vi "roboRIO v1.0 Reserve Timer IRQ.vi"(4 "Callback VI Ref":T1, 5 "Allow Overwrite?":bool, 7 "Reserve?":bool, 8 "error in (no error)":errorcluster, 10 "Interval(us)":u32, 11 "Timer ID":u8) -> (0 "error out":errorcluster, 2 "Succeed?":bool)   [LabVIEW 2021]
uses:
  <vilib>/myRIO/Common/Instrument Driver Framework/myRIO v1.0/IRQ/typedefs/Callback VI Ref.ctl
  <vilib>/myRIO/Common/Instrument Driver Framework/Utilities/typedefs/FPGA Ref Manager Action Enum.ctl
  <vilib>/myRIO/Common/Instrument Driver Framework/myRIO v1.0/IRQ/typedefs/Timer IRQ.ctl
  <vilib>/myRIO/Common/Instrument Driver Framework/myRIO v1.0/IRQ/typedefs/IO IRQ Channels Enum.ctl
  <vilib>/myRIO/Common/Instrument Driver Framework/myRIO v1.0/IRQ/typedefs/IRQ Type.ctl
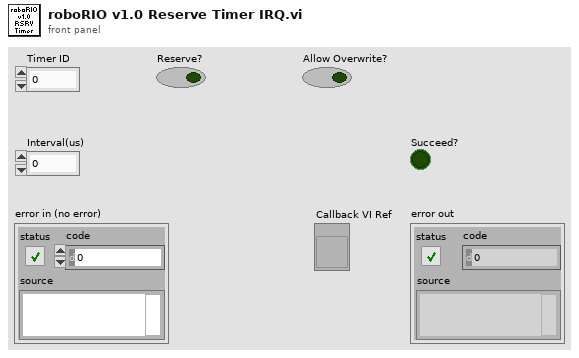
[diagram p1: front panel]
types:
  T1 = typedef "Callback VI Ref.ctl" = refnum<vi>
  T2 = typedef "FPGA Ref Manager Action Enum.ctl" = enum16{"Get", "Set", "Reset"}
  T3 = typedef "Timer IRQ.ctl" = cluster{"Remaining(us)":u32, "Timer ID":u8, "Interval(us)":u32, "Callback VI Ref":T1, "Allow Overwrite?":bool, "Timer enabled?":bool}
  T4 = typedef "IO IRQ Channels Enum.ctl" = enum16{"Not Connected", "A/AI0 (Interrupt)", "A/AI1 (Interrupt)", "A/DIO0 (Interrupt)", "A/DIO1 (Interrupt)", "A/DIO2 (Interrupt)", "A/DIO3 (Interrupt)", "Button0 (Interrupt)", "B/AI0 (Interrupt)", "B/AI1 (Interrupt)", "B/DIO0 (Interrupt)", "B/DIO1 (Interrupt)", "B/DIO2 (Interrupt)", "B/DIO3 (Interrupt)"}
  T5 = typedef "IRQ Type.ctl" = enum16{"Timer", "Analog falling edge", "Analog rising edge", "Digital falling edge", "Digital rising edge", "Digital edge"}
  T6 = typedef "Timer IRQ Array.ctl" = T3[]
  T7 = typedef "Generic FPGA Reference.ctl" = refnum<k20>
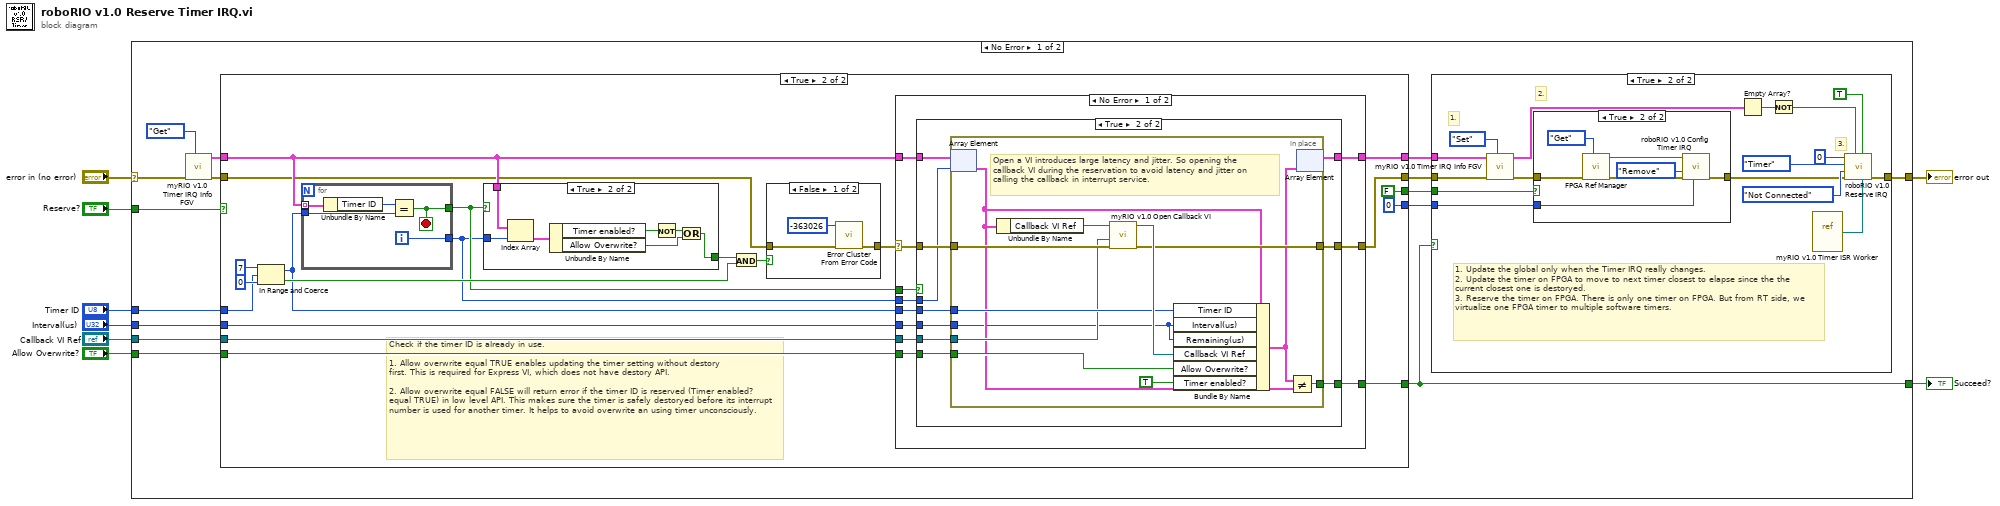
[diagram p0: block diagram]
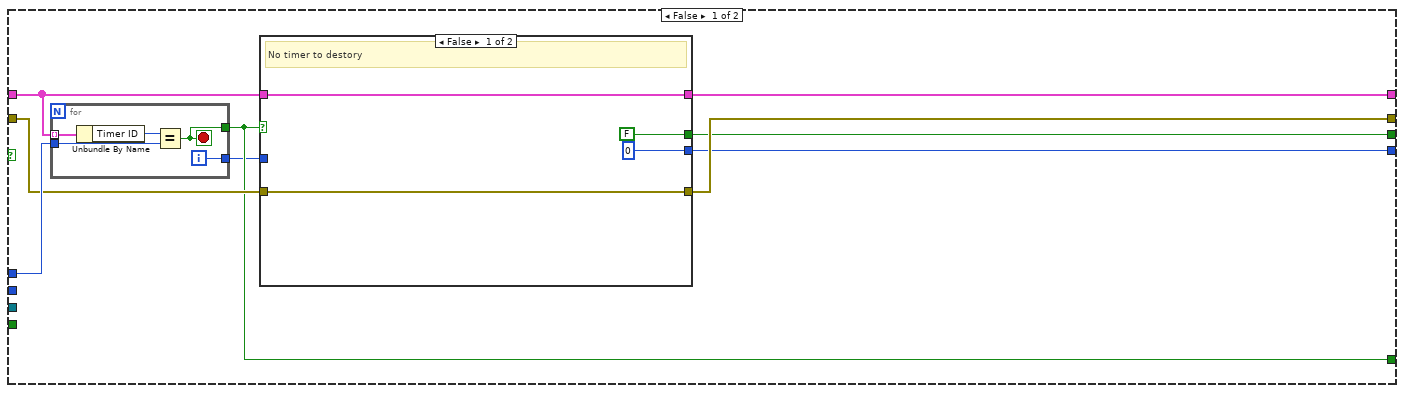
[diagram p2: hidden frame]
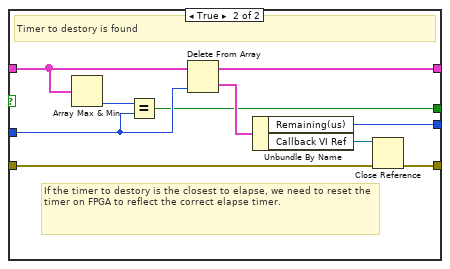
[diagram p3: hidden frame]
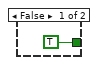
[diagram p4: hidden frame]
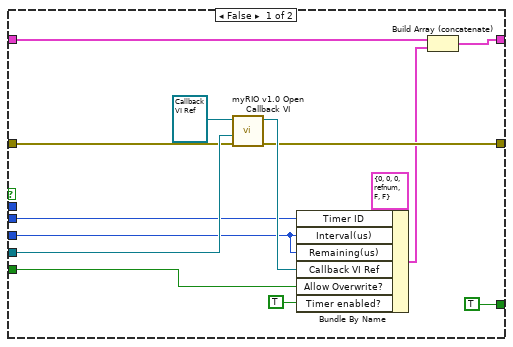
[diagram p6: hidden frame]
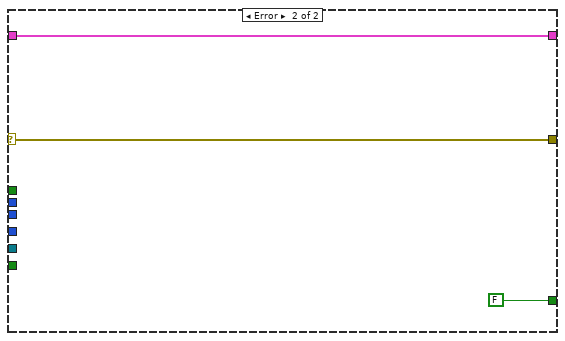
[diagram p7: hidden frame]
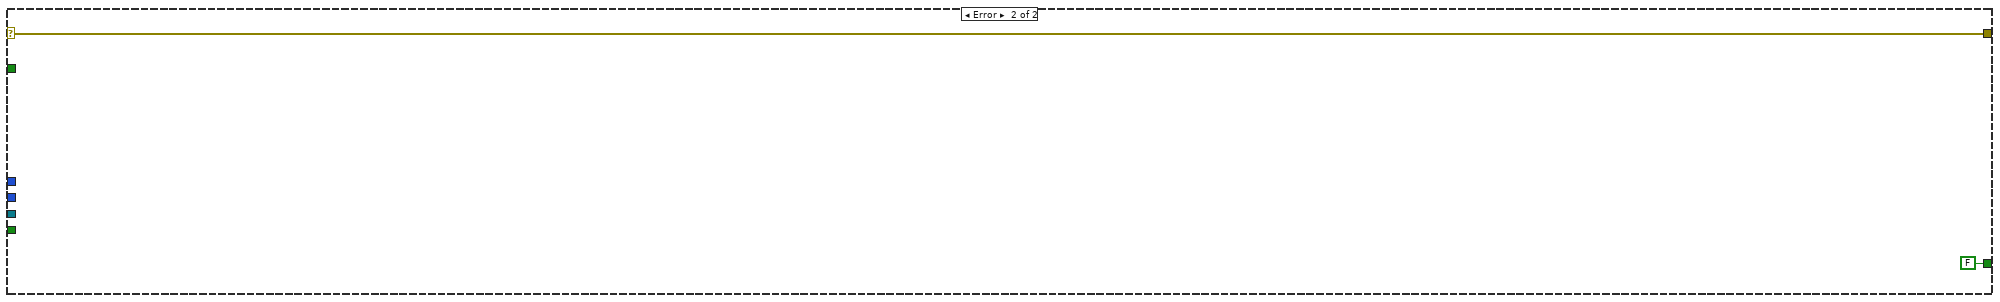
[diagram p10: hidden frame]
diagram:
  n1 = case shown="No Error" "error in (no error)" {
    selector: "error in (no error)" -> [w9 w165]
    tunnel: "Callback VI Ref" -> [w23 _]
    tunnel: [w21 w165] -> w7
    tunnel: "Allow Overwrite?" -> [w20 _]
    tunnel: "Interval(us)" -> [w19 _]
    tunnel: "Timer ID" -> [w16 _]
    tunnel: [w14 FALSE] -> w3
    tunnel: "Reserve?" -> [w12 _]
    frame No Error {
      n2 = call <vilib>:"myRIO v1.0 Timer IRQ Info FGV.vi"("Action"=FPGA_Ref_Manager_Action_Enum."Get", "error in (no error)"=w9) -> ("error out"=w13:errorcluster, "Timer IRQ Array out"=w17:T6)  [unwired: 8 in]
      n3 = case shown="True" w12 {
        tunnel: w23 -> [_ w71]
        tunnel: [w28 w70] -> w22
        tunnel: w20 -> [_ w69]
        tunnel: w19 -> [_ w68]
        tunnel: w17 -> [w32 w62]
        tunnel: w16 -> [w31 w61]
        tunnel: [w27 w56] -> w15
        tunnel: [w29 w55] -> w14
        tunnel: w13 -> [w30 w54]
        tunnel: [w25 FALSE] -> w11
        tunnel: [w24 u32 0 ("Remaining(us)")] -> w10
        frame False {
          n4 = for {
            tunnel: w32 -> [w51] mode=indexing
            tunnel: w31 -> [w49]
            tunnel: [w48] -> w29
            tunnel: [w47] -> w26
            i -> [w47]
            stop <- w48 stop-if-true
            n5 = Unbundle By Name(w51) -> ("Timer ID"=w50:u8)
            n6 = Equal?(x=w50, y=w49) -> (x = y?=w48:bool)
          }
          n7 = case shown="False" w29 {
            tunnel: w32 -> [w35 w44]
            tunnel: w30 -> [w36 w41]
            tunnel: [w36 w39] -> w27
            tunnel: [w35 w40] -> w28
            tunnel: w26 -> [_ w43]
            tunnel: [FALSE w38] -> w25
            tunnel: [u32 0 ("Remaining(us)") w37] -> w24
            frame False {
              # "No timer to destory"
            }
            frame True {
              # "If the timer to destory is the closest to elapse, we need to reset the timer on FPGA to reflect the correct elapse timer."
              # "Timer to destory is found"
              n8 = Array Max & Min(array=w44) -> (min index (indices)=w46:i32)  [unwired: 3 out]
              n9 = Equal?(x=w46, y=w43) -> (x = y?=w38:bool)
              n10 = Delete From Array(array=w44, index=w43) -> (deleted portion=w45:T3, array with subset deleted=w40:T6)  [unwired: 1 in]
              n11 = Unbundle By Name(w45) -> ("Remaining(us)"=w37:u32, "Callback VI Ref"=w42:T1)
              n12 = Close Reference(reference=w42, error in (no error)=w41) -> (error out=w39:errorcluster)
            }
          }
        }
        frame True {
          # "Check if the timer ID is already in use.\n\n1. Allow overwrite equal TRUE enables updating the timer setting without destory\nfirst. This is required for Express VI, which does not have destory API.\n\n2. Allow overwrite equal FALSE will return error if the timer ID is reserved (Timer enabled? equal TRUE) in low level API. This makes sure the timer is safely destoryed before its interrupt number is used for another timer. It helps to avoid overwrite an using timer unconsciously."
          n13 = In Range and Coerce(upper limit=u8 7, x=w61, lower limit=u8 0) -> (coerced(x)=w60:u8, In Range?=w65:bool)
          n14 = for {
            tunnel: w62 -> [w88] mode=indexing
            tunnel: w60 -> [w86]
            tunnel: [w85] -> w59
            tunnel: [w84] -> w58
            i -> [w84]
            stop <- w85 stop-if-true
            n15 = Unbundle By Name(w88) -> ("Timer ID"=w87:u8)
            n16 = Equal?(x=w87, y=w86) -> (x = y?=w85:bool)
          }
          n17 = case shown="True" w59 {
            tunnel: w62 -> [_ w79]
            tunnel: w58 -> [_ w78]
            tunnel: [TRUE w76] -> w66
            frame False {
            }
            frame True {
              n18 = Index Array(array=w79, index=w78) -> (element=w77:T3)
              n19 = Unbundle By Name(w77) -> ("Timer enabled?"=w74:bool, "Allow Overwrite?"=w73:bool)
              n20 = Not(x=w74) -> (.not. x?=w75:bool)
              n21 = Or(x=w75, y=w73) -> (x .or. y?=w76:bool)
            }
          }
          n22 = And(x=w66, y=w65) -> (x .and. y?=w67:bool)
          n23 = case shown="False" w67 {
            tunnel: [w81 w83] -> w57
            tunnel: w54 -> [w80 w83]
            frame False {
              n24 = call <vilib>:"Error Cluster From Error Code.vi"("error in (no error)"=w80, "error code (0)"=-363026) -> ("error out"=w81:errorcluster)  [unwired: 7 in]
            }
            frame True {
            }
          }
          n25 = case shown="No Error" w57 {
            selector: w57 -> [w97 w137]
            tunnel: w71 -> [w94 _]
            tunnel: w60 -> [w95 _]
            tunnel: w62 -> [w93 w138]
            tunnel: w58 -> [w91 _]
            tunnel: [w92 w138] -> w70
            tunnel: w69 -> [w99 _]
            tunnel: w68 -> [w98 _]
            tunnel: w59 -> [w90 _]
            tunnel: [w96 w137] -> w56
            tunnel: [w89 FALSE] -> w55
            frame No Error {
              n26 = case shown="True" w90 {
                tunnel: w99 -> [w103 w123]
                tunnel: w98 -> [w100 w122]
                tunnel: w97 -> [w107 w121]
                tunnel: [w106 w120] -> w96
                tunnel: w95 -> [w104 w119]
                tunnel: w94 -> [w109 w118]
                tunnel: w93 -> [w113 w117]
                tunnel: [w112 w116] -> w92
                tunnel: w91 -> [_ w115]
                tunnel: [TRUE w114] -> w89
                frame False {
                  n27 = call <vilib>:"myRIO v1.0 Open Callback VI.vi"("error in (no error)"=w107, "Static Ref in"=w109, "Opened VI Ref in"=T1 refnum) -> ("error out"=w106:errorcluster, "Opened VI Ref out"=w108:T1)  [unwired: 7 in]
                  n28 = Bundle By Name(cluster=T3 {"Remaining(us)"=0, "Timer ID"=0, "Interval(us)"=0, "Callback VI Ref"=refnum, "Allow Overwrite?"=FALSE, "Timer enabled?"=FALSE} ("Interrupt Info"), "Timer ID"=w104, "Interval(us)"=w100, "Remaining(us)"=w100, "Callback VI Ref"=w108, "Allow Overwrite?"=w103, "Timer enabled?"=TRUE ("Timer used?")) -> (w105:T3)
                  n29 = Build Array (concatenate)(w113, w105) -> (w112:T6)
                }
                frame True {
                  n30 = in-place {
                    in-place-border: w123 -> [w134]
                    in-place-border: w122 -> [w124]
                    in-place-border: w121 -> [w132]
                    in-place-border: [w131] -> w120
                    in-place-border: w119 -> [w130]
                    in-place-border: w118 -> [w128]
                    in-place-border: [w126] -> w114
                    # "Open a VI introduces large latency and jitter. So opening the callback VI during the reservation to avoid latency and jitter on calling the callback in interrupt service."
                    n31 = in-place-array #1(w117, w115) -> (w125:T3)
                    n32 = Unbundle By Name(w125) -> ("Callback VI Ref"=w129:T1)
                    n33 = call <vilib>:"myRIO v1.0 Open Callback VI.vi"("error in (no error)"=w132, "Static Ref in"=w128, "Opened VI Ref in"=w129) -> ("error out"=w131:errorcluster, "Opened VI Ref out"=w133:T1)  [unwired: 7 in]
                    n34 = Bundle By Name(cluster=w125, "Timer ID"=w130, "Interval(us)"=w124, "Remaining(us)"=w124, "Callback VI Ref"=w133, "Allow Overwrite?"=w134, "Timer enabled?"=TRUE ("Timer used?")) -> (w127:T3)
                    n35 = Not Equal?(x=w127, y=w125) -> (x != y?=w126:bool)
                    n36 = in-place-array #1(w127) -> (w116:T6)  [unwired: 1 out]
                  }
                }
              }
            }
            frame Error {
            }
          }
        }
      }
      n37 = case shown="True" w14 {
        tunnel: w22 -> [_ w153]
        tunnel: [w139 w144] -> w21
        tunnel: w15 -> [w139 w154]
        tunnel: w11 -> [_ w143]
        tunnel: w10 -> [_ w142]
        frame False {
        }
        frame True {
          # "3."
          # "2."
          # "1."
          # "1. Update the global only when the Timer IRQ really changes.\n2. Update the timer on FPGA to move to next timer closest to elapse since the the current closest one is destoryed.\n3. Reserve the timer on FPGA. There is only one timer on FPGA. But from RT side, we virtualize one FPGA timer to multiple software timers."
          n38 = call <vilib>:"myRIO v1.0 Timer IRQ Info FGV.vi"("Action"=FPGA_Ref_Manager_Action_Enum."Set", "error in (no error)"=w154, "Timer IRQ Array in"=w153) -> ("error out"=w141:errorcluster, "Timer IRQ Array out"=w145:T6)  [unwired: 7 in]
          n39 = case shown="True" w143 {
            tunnel: w142 -> [_ w159]
            tunnel: w141 -> [w156 w158]
            tunnel: [w156 w157] -> w140
            frame False {
            }
            frame True {
              n40 = call <vilib>:"FPGA Ref Manager.vi"("Action"=FPGA_Ref_Manager_Action_Enum."Get", "error in (no error)"=w158) -> ("error out"=w162:errorcluster, "Generic FPGA Reference out"=w163:T7)  [unwired: 7 in]
              n41 = call <vilib>:"roboRIO v1.0 Config Timer IRQ.vi"("Remaining Time"=w159, "error in (no error)"=w162, "Action"=enum16{"Add", "Update", "Remove"}."Remove", "myRIO FPGA Ref In"=w163) -> ("error out"=w157:errorcluster)  [unwired: 5 in, 2 out]
            }
          }
          n42 = Empty Array?(array=w145) -> (empty?=w151:bool)
          n43 = Not(x=w151) -> (.not. x?=w150:bool)
          n44 = vi-ref <vilib>:"myRIO v1.0 Timer ISR Worker.vi"() -> ("vi reference"=w146:refnum<vi>)
          n45 = call <vilib>:"roboRIO v1.0 Reserve IRQ.vi"("Callback VI Ref"=w146, "Allow Overwrite? (F)"=TRUE, "Is Reserve?"=w150, "error in (no error)"=w140, "IO IRQ Channels Enum"=IO_IRQ_Channels_Enum."Not Connected", "IRQ Type"=IRQ_Type."Timer", "IRQ Number"=u8 0) -> ("error out"=w144:errorcluster)  [unwired: 3 in, 1 out]
        }
      }
    }
    frame Error {
    }
  }
  "error out" <- w7
  "Succeed?" <- w3
